vi "GUI_v3.vi"() -> ()   [LabVIEW 2023]
uses:
  Serial - Settings.ctl
  <vilib>/Utility/miscctls.llb/LVRGBAColorTypeDef.ctl
  <vilib>/Utility/miscctls.llb/LV3DPointTypeDef.ctl
  e2109eba-4716-5941-afb7-b0faa504542a.vi
  327bca25-9371-1e41-8126-f95c64e27f6d.vi
  abf5b892-6ba6-6f43-be19-45be42e399fc.vi
  44eb8c8b-3870-a84c-bb75-4112acaa9c04.vi
  f7abd40d-e190-3443-8a30-185c2517432b.vi
  <vilib>/Array/Sort 2D Array - Pop Stack.vi
  <vilib>/Array/Sort 2D Array - Push Stack.vi
  327bca25-9371-1e41-8126-f95c64e27f6d.vi/269d4b3b-47f5-49e3-8884-44851e4dd9d5.vi
  327bca25-9371-1e41-8126-f95c64e27f6d.vi/6d99389c-673d-4efb-bf33-19b32bcf4cf8.vi
  abf5b892-6ba6-6f43-be19-45be42e399fc.vi/269d4b3b-47f5-49e3-8884-44851e4dd9d5.vi
  abf5b892-6ba6-6f43-be19-45be42e399fc.vi/6d99389c-673d-4efb-bf33-19b32bcf4cf8.vi
  44eb8c8b-3870-a84c-bb75-4112acaa9c04.vi/269d4b3b-47f5-49e3-8884-44851e4dd9d5.vi
  44eb8c8b-3870-a84c-bb75-4112acaa9c04.vi/6d99389c-673d-4efb-bf33-19b32bcf4cf8.vi
  f7abd40d-e190-3443-8a30-185c2517432b.vi/269d4b3b-47f5-49e3-8884-44851e4dd9d5.vi
  f7abd40d-e190-3443-8a30-185c2517432b.vi/6d99389c-673d-4efb-bf33-19b32bcf4cf8.vi
  <vilib>/Instr/_visa.llb/VISA Configure Serial Port (Instr).vi
  <vilib>/picture/3D Picture Control/Object/Create Object (drawable).vi
  <vilib>/picture/3D Picture Control/Object/Add Object (no reference).vi
  <vilib>/picture/3D Picture Control/NI_3D Picture Control.lvlib
panel:
  out "read buffer":string
  out "output string":string
  in  "X":bool
  in  "Y":bool
  in  "Z":bool
  in  "[ESC]":bool
  out "Buffer length":i32
  in  "Serial Settings":T1={"baud rate"=115200, "data bits"=8, "parity"=enum."None", "stop bits"=10, "flow control"=0} {"flow control" items=["None"=0, "XON/XOFF"=1, "RTS/CTS"=2, "DTR/DSR"=4]; "stop bits" items=["1.0"=10, "1.5"=15, "2.0"=20]; "data bits" min=5 max=8 step=1; "baud rate" items=["75"=75, "110"=110, "134"=134, "150"=150, "300"=300, "600"=600, "1200"=1200, "1800"=1800, "2400"=2400, "4800"=4800, "7200"=7200, "9600"=9600, "14400"=14400, "19200"=19200, "28800"=28800, "38400"=38400, "56000"=56000, "57600"=57600, "115200"=115200, "128000"=128000, "230400"=230400]}
  out "Input length":i32
  in  "Draw Mode":T2(ring)
  in  "Front":bool
  out "3D Picture":refnum<vi>(3d-picture)
  out "Number of Points":i32
  in  "Clear":bool
  in  "From File?":bool
  in  "File path":path
  in  "VISA resource name":refnum<visa-resource-name>
  in  "Back":bool
  in  "Up":bool
  in  "Down":bool
  in  "Right":bool
  in  "Left":bool
  # "3D LED HOLOGRAM\n1. Enter VISA resource name\n2. Import a file\n3. Run the program"
  # "FIVE GUYS"
  # "Import File"
  # "TRANSLATION"
  # "X"
  # "Y"
  # "Z"
  # "ROTATION"
  # "X"
  # "Y"
  # "Z"
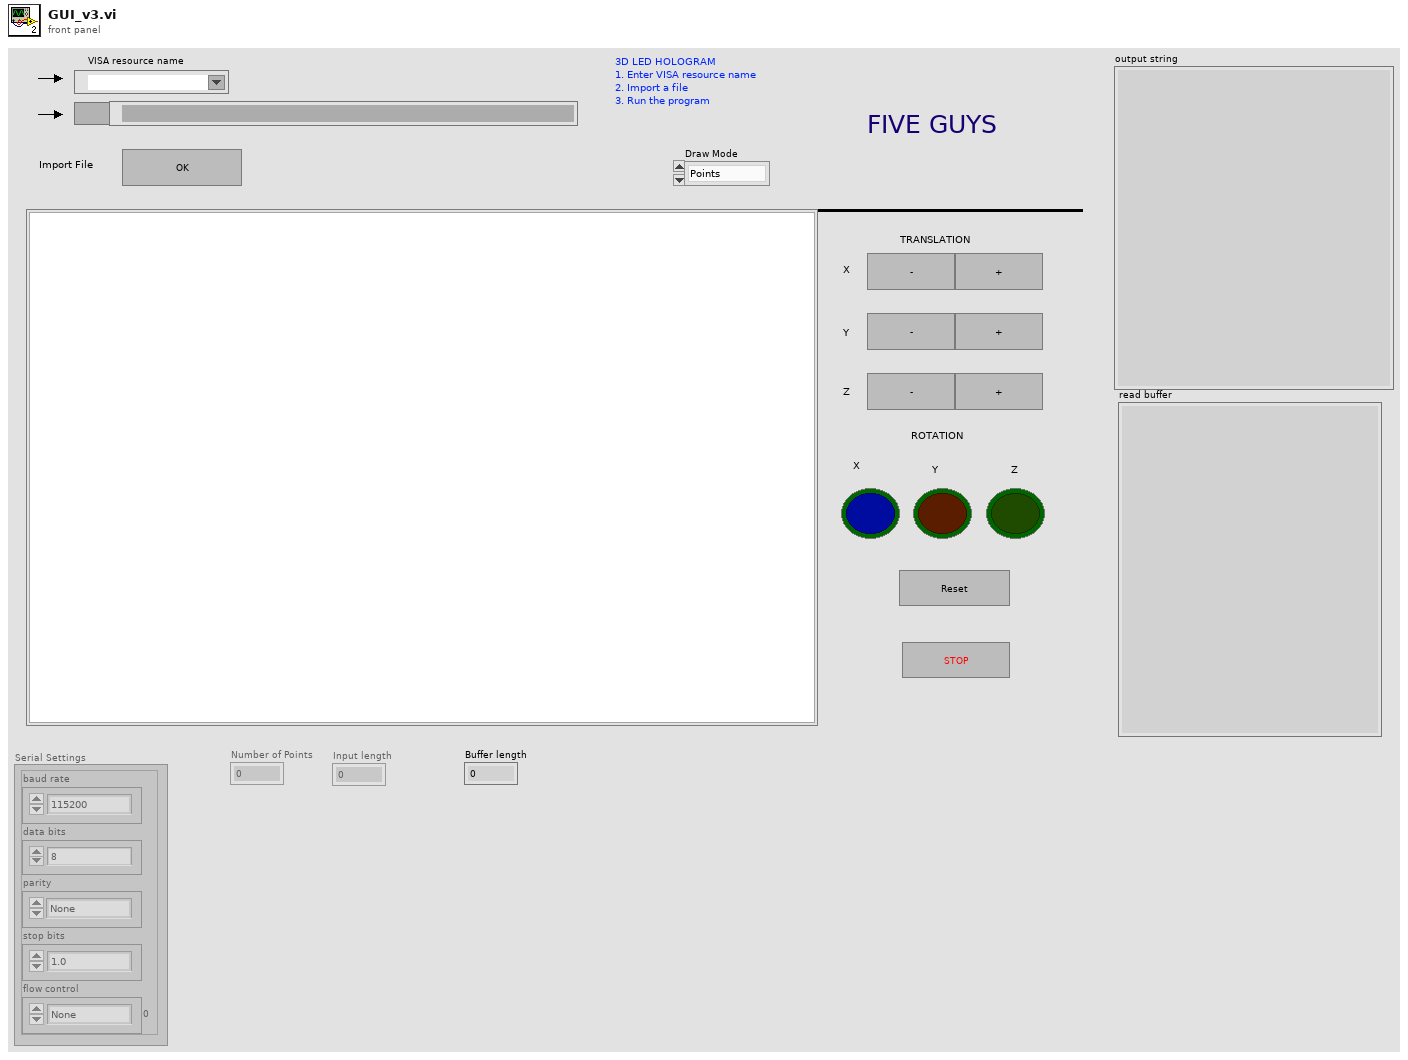
[diagram p1: front panel]
types:
  T1 = typedef "Serial - Settings.ctl" = cluster{"baud rate":u32, "data bits":u16, "parity":enum16{"None", "Odd", "Even", "Mark", "Space"}, "stop bits":u16, "flow control":u16}
  T2 = enum16{"Points", "Lines", "Line Strip", "Line Loop", "Triangles", "Triangle Strip", "Triangle Fan", "Quads", "Quad Strip", "Polygon"}
  T3 = typedef "LVRGBAColorTypeDef.ctl" = cluster{"Red":sgl, "Green":sgl, "Blue":sgl, "Alpha":sgl}
  T4 = enum16{"Overall", "Per Primitive", "Per Vertex", "Binding Off"}
  T5 = cluster{"Red":sgl, "Green":sgl, "Blue":sgl, "Alpha":sgl}
  T6 = typedef "LV3DPointTypeDef.ctl" = cluster{"X":sgl, "Y":sgl, "Z":sgl}
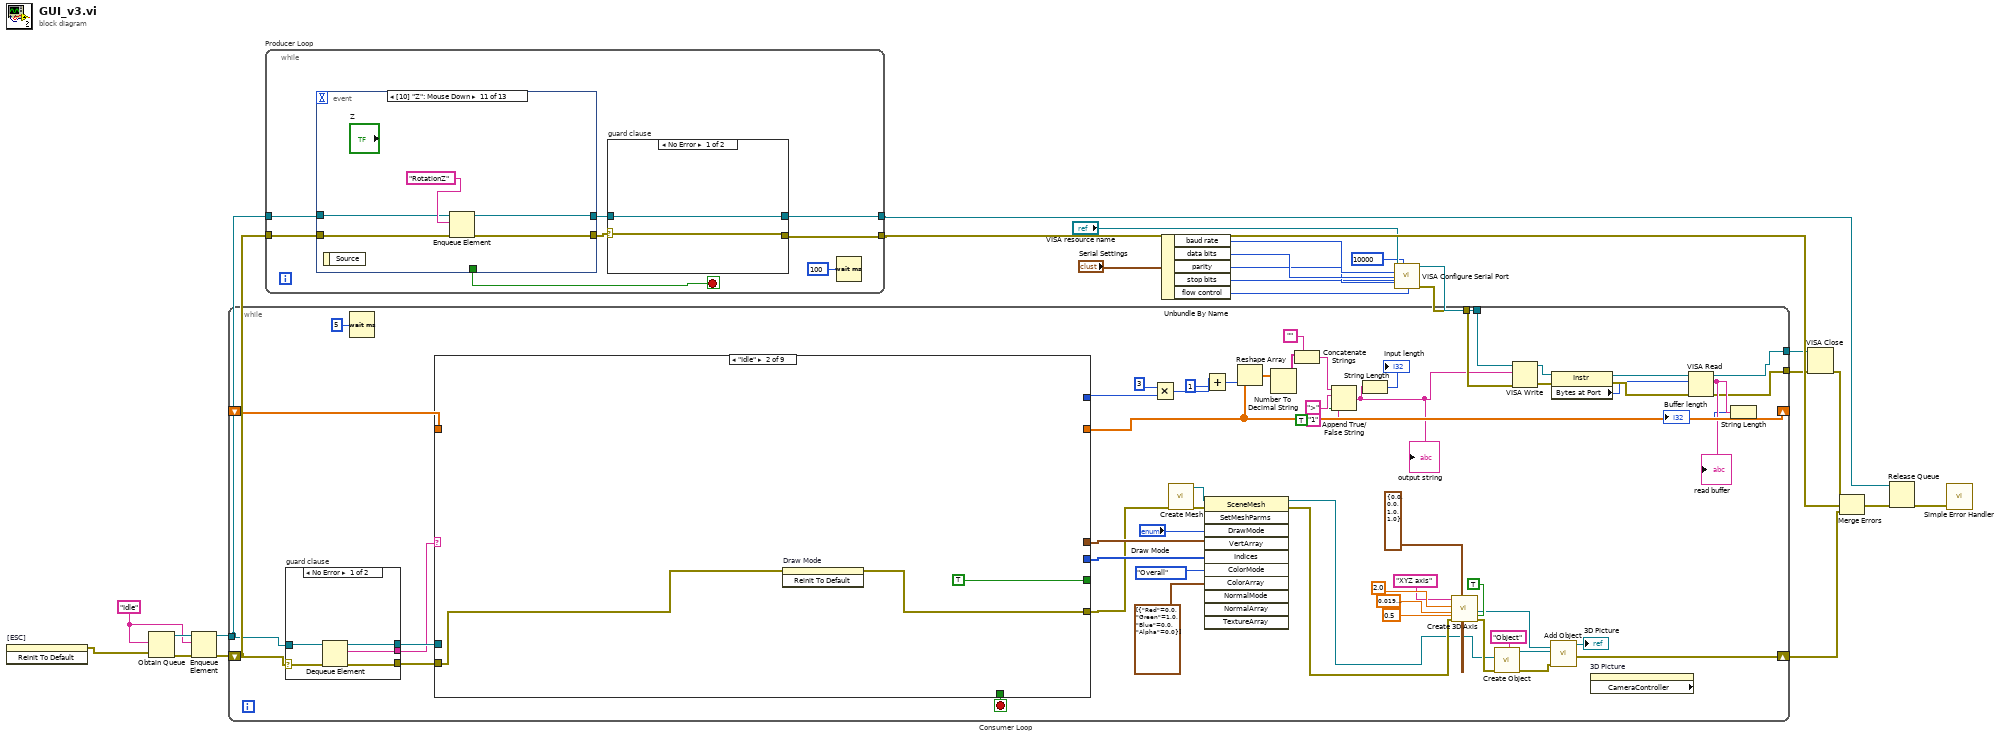
[diagram p0: block diagram]
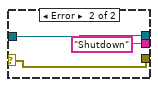
[diagram p2: hidden frame]
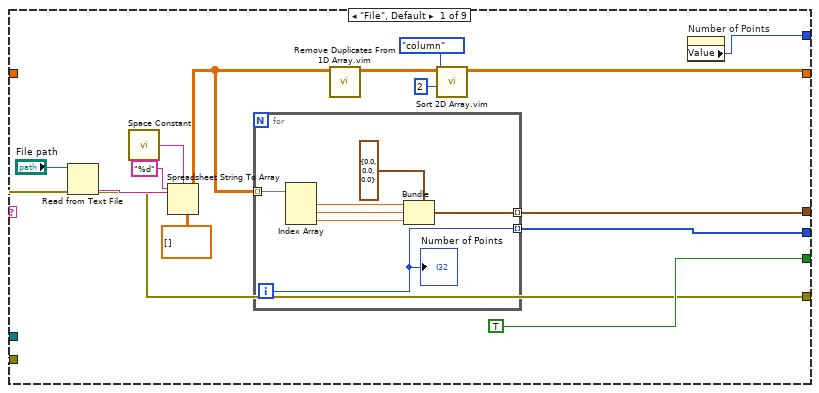
[diagram p3: hidden frame]
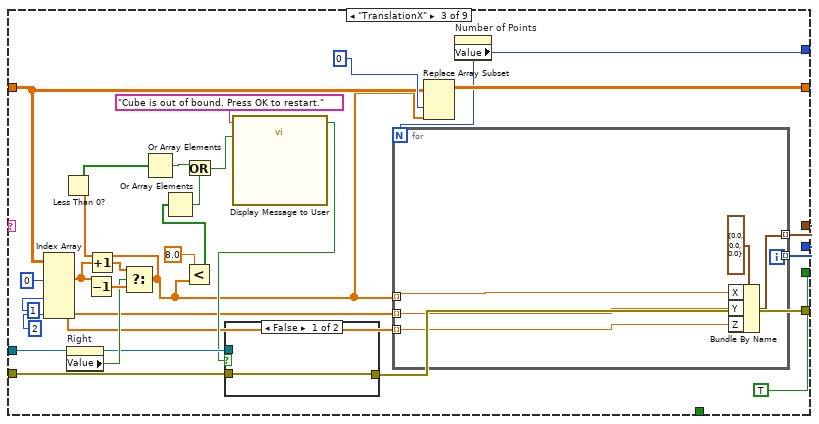
[diagram p4: hidden frame]
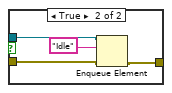
[diagram p5: hidden frame]
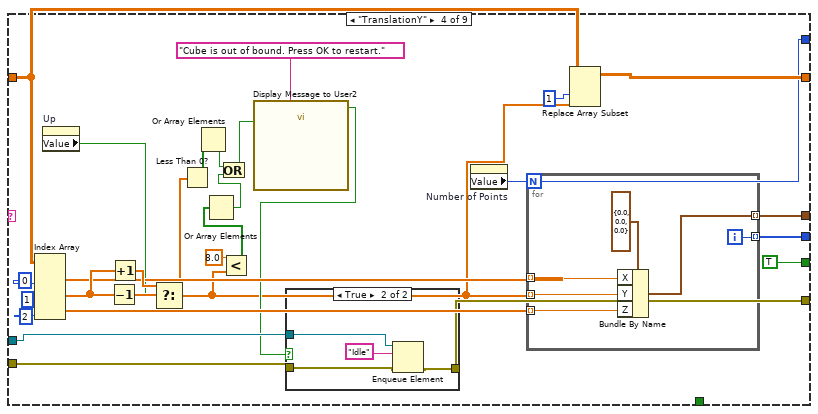
[diagram p6: hidden frame]
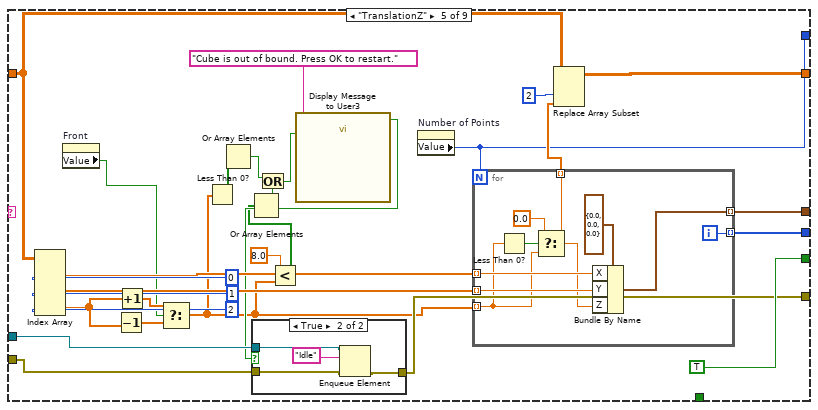
[diagram p8: hidden frame]
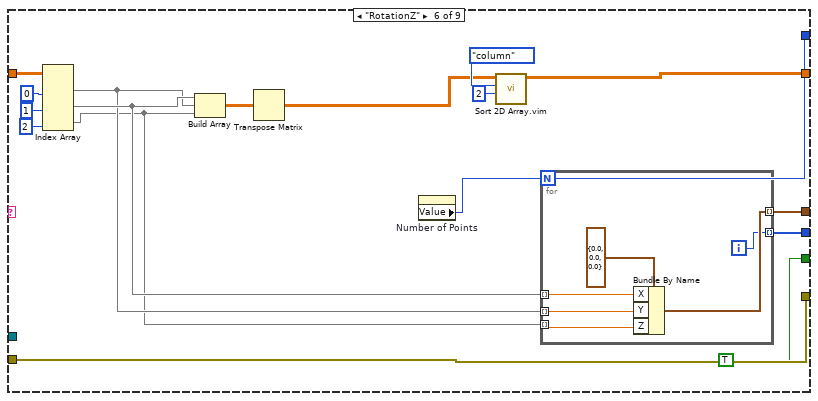
[diagram p10: hidden frame]
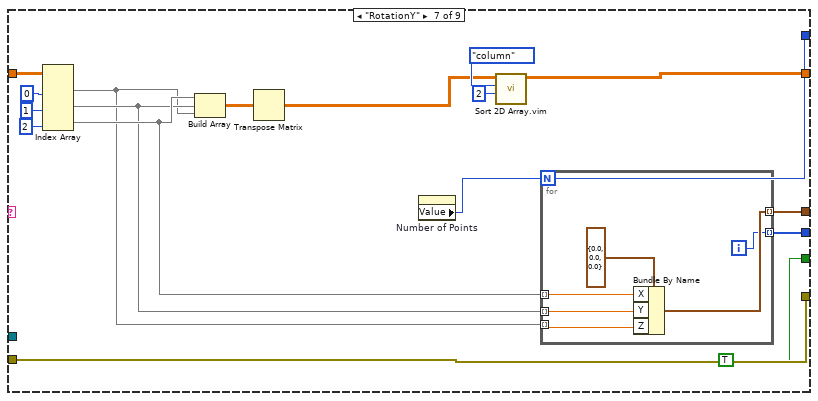
[diagram p11: hidden frame]
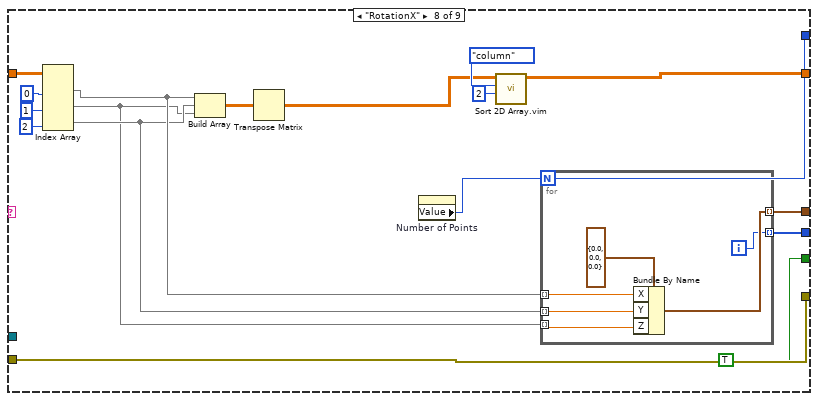
[diagram p12: hidden frame]
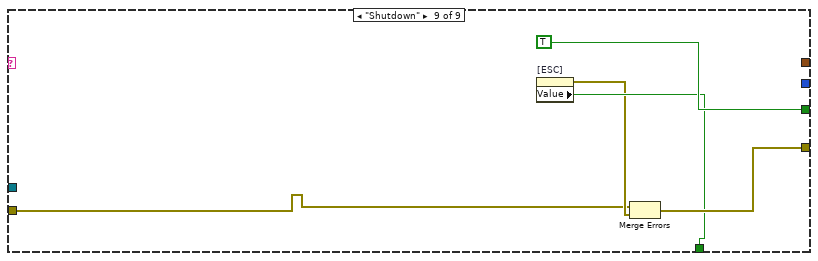
[diagram p13: hidden frame]
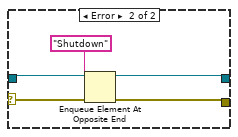
[diagram p14: hidden frame]
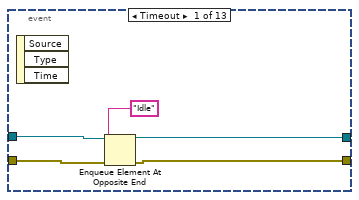
[diagram p15: hidden frame]
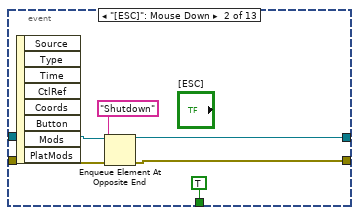
[diagram p16: hidden frame]
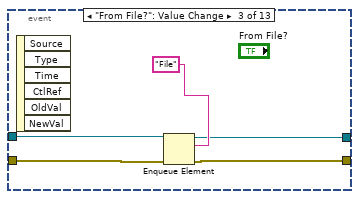
[diagram p17: hidden frame]
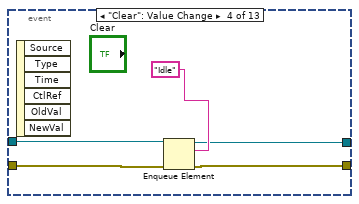
[diagram p18: hidden frame]
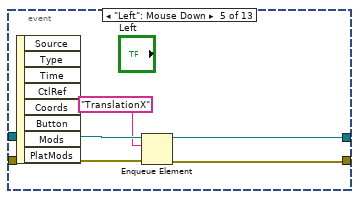
[diagram p19: hidden frame]
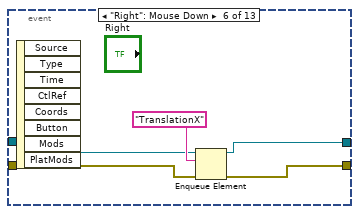
[diagram p20: hidden frame]
diagram:
  w22 = "Idle"
  n1 = invoke on="[ESC]" class="Bool (strict)" method="Reinit To Default"() -> (error out=w1:errorcluster)  [unwired: 3 in, 2 out]
  n2 = Obtain Queue(element data type=w22, error in (no error)=w1) -> (queue out=w23:refnum<queue>, error out=w24:errorcluster)  [unwired: 3 in, 1 out]
  n3 = Enqueue Element(queue=w23, element=w22, error in (no error)=w24) -> (queue out=w21:refnum<queue>, error out=w20:errorcluster)  [unwired: 1 in, 1 out]
  n4 = while "Producer Loop" {
    tunnel: [w28] -> w17
    tunnel: [w27] -> w19
    tunnel: w21 -> [w32]
    tunnel: w20 -> [w31]
    stop <- w26 stop-if-true
    n5 = event shown="[10] \"Z\": Mouse Down" {
      selector: _ -> [_ _ _ _ _ _ _ _ _ _ _ _ _]
      dyn-events: _ -> [_ _ _ _ _ _ _ _ _ _ _ _ _]
      timeout: _ -> [_ _ _ _ _ _ _ _ _ _ _ _ _]
      tunnel: [_ TRUE ("[ESC]") _ _ _ _ _ _ _ _ _ _ _] -> w26
      tunnel: [w43 w49 w51 w56 w61 w66 w71 w76 w81 w86 w94 w99 w104] -> w29
      tunnel: [w42 w48 w52 w57 w64 w67 w72 w77 w82 w87 w93 w98 w103] -> w30
      tunnel: w32 -> [w41 w47 w53 w58 w65 w69 w74 w79 w84 w89 w92 w97 w102]
      tunnel: w31 -> [w40 w46 w54 w59 w63 w68 w73 w78 w83 w88 w91 w96 w101]
      event Timeout {
        n6 = event-data() -> ()  [unwired: 1 in, 3 out]
        n7 = Enqueue Element At Opposite End(queue=w41, element="Idle", error in (no error)=w40) -> (queue out=w42:refnum<queue>, error out=w43:errorcluster)  [unwired: 1 in, 1 out]
      }
      event "[ESC]": Mouse Down {
        n8 = event-data() -> ()  [unwired: 1 in, 8 out]
        n9 = Enqueue Element At Opposite End(queue=w47, element="Shutdown", error in (no error)=w46) -> (queue out=w48:refnum<queue>, error out=w49:errorcluster)  [unwired: 1 in, 1 out]
      }
      event "From File?": Value Change {
        n10 = event-data() -> ()  [unwired: 1 in, 6 out]
        n11 = Enqueue Element(queue=w53, element="File", error in (no error)=w54) -> (queue out=w52:refnum<queue>, error out=w51:errorcluster)  [unwired: 1 in, 1 out]
      }
      event "Clear": Value Change {
        n12 = event-data() -> ()  [unwired: 1 in, 6 out]
        n13 = Enqueue Element(queue=w58, element="Idle", error in (no error)=w59) -> (queue out=w57:refnum<queue>, error out=w56:errorcluster)  [unwired: 1 in, 1 out]
      }
      event "Left": Mouse Down {
        n14 = event-data() -> ()  [unwired: 1 in, 8 out]
        n15 = Enqueue Element(queue=w65, element="TranslationX", error in (no error)=w63) -> (queue out=w64:refnum<queue>, error out=w61:errorcluster)  [unwired: 1 in, 1 out]
      }
      event "Right": Mouse Down {
        n16 = event-data() -> ()  [unwired: 1 in, 8 out]
        n17 = Enqueue Element(queue=w69, element="TranslationX", error in (no error)=w68) -> (queue out=w67:refnum<queue>, error out=w66:errorcluster)  [unwired: 1 in, 1 out]
      }
      event "Back": Mouse Down {
        n18 = event-data() -> ()  [unwired: 1 in, 8 out]
        n19 = Enqueue Element(queue=w74, element="TranslationZ", error in (no error)=w73) -> (queue out=w72:refnum<queue>, error out=w71:errorcluster)  [unwired: 1 in, 1 out]
      }
      event "Front": Mouse Down {
        n20 = event-data() -> ()  [unwired: 1 in, 8 out]
        n21 = Enqueue Element(queue=w79, element="TranslationZ", error in (no error)=w78) -> (queue out=w77:refnum<queue>, error out=w76:errorcluster)  [unwired: 1 in, 1 out]
      }
      event "Down": Mouse Down {
        n22 = event-data() -> ()  [unwired: 1 in, 8 out]
        n23 = Enqueue Element(queue=w84, element="TranslationY", error in (no error)=w83) -> (queue out=w82:refnum<queue>, error out=w81:errorcluster)  [unwired: 1 in, 1 out]
      }
      event "Up": Mouse Down {
        n24 = event-data() -> ()  [unwired: 1 in, 8 out]
        n25 = Enqueue Element(queue=w89, element="TranslationY", error in (no error)=w88) -> (queue out=w87:refnum<queue>, error out=w86:errorcluster)  [unwired: 1 in, 1 out]
      }
      event "Z": Mouse Down {
        n26 = event-data() -> ()  [unwired: 1 in, 1 out]
        n27 = Enqueue Element(queue=w92, element="RotationZ", error in (no error)=w91) -> (queue out=w93:refnum<queue>, error out=w94:errorcluster)  [unwired: 1 in, 1 out]
      }
      event "Y": Mouse Down {
        n28 = event-data() -> ()  [unwired: 1 in, 1 out]
        n29 = Enqueue Element(queue=w97, element="RotationY", error in (no error)=w96) -> (queue out=w98:refnum<queue>, error out=w99:errorcluster)  [unwired: 1 in, 1 out]
      }
      event "X": Mouse Down {
        n30 = event-data() -> ()  [unwired: 1 in, 1 out]
        n31 = Enqueue Element(queue=w102, element="RotationX", error in (no error)=w101) -> (queue out=w103:refnum<queue>, error out=w104:errorcluster)  [unwired: 1 in, 1 out]
      }
    }
    n32 = case "guard clause" shown="No Error" w29 {
      selector: w29 -> [w33 w38]
      tunnel: w30 -> [w34 w39]
      tunnel: [w34 w36] -> w28
      tunnel: [w33 w37] -> w27
      frame No Error {
      }
      frame Error {
        n33 = Enqueue Element At Opposite End(queue=w39, element="Shutdown", error in (no error)=w38) -> (queue out=w36:refnum<queue>, error out=w37:errorcluster)  [unwired: 1 in, 1 out]
      }
    }
    n34 = Wait (ms)(milliseconds to wait=u32 100) -> ()  [unwired: 1 out]
  }
  n35 = Unbundle By Name("Serial Settings") -> ("baud rate"=w10:u32, "data bits"=w9:u16, "parity"=w8:enum16{"None", "Odd", "Even", "Mark", "Space"}, "stop bits"=w7:u16, "flow control"=w6:u16)
  n36 = call-poly "VISA Configure Serial Port"("VISA resource name"="VISA resource name", "timeout (10sec)"=u32 10000, "baud rate (9600)"=w10, "data bits (8)"=w9, "parity (0:none)"=w8, "stop bits (10: 1 bit)"=w7, "flow control (0:none)"=w6) -> ("VISA resource name out"=w5:refnum<visa-resource-name>, "error out"=w4:errorcluster)  [unwired: 7 in]
  n37 = while "Consumer Loop" {
    tunnel: w21 -> [w162]
    shift-right: [w135] -> w16
    shift-left: w20 -> [w159]
    shift-right: [w134] -> _
    shift-left: _ -> [w156]
    tunnel: w5 -> [w144]
    tunnel: w4 -> [w143]
    tunnel: [w106] -> w15
    tunnel: [w107] -> w14
    stop <- w160 stop-if-true
    n38 = case "guard clause" shown="No Error" w159 {
      selector: w159 -> [w166 w169]
      tunnel: w162 -> [w167 w170]
      tunnel: [w165 w169] -> w161
      tunnel: [w164 "Shutdown"] -> w117
      tunnel: [w163 w170] -> w142
      frame No Error {
        n39 = Dequeue Element(queue=w167, error in (no error)=w166) -> (queue out=w163:refnum<queue>, element=w164:string, error out=w165:errorcluster)  [unwired: 1 in, 1 out]
      }
      frame Error {
      }
    }
    n40 = Wait (ms)(milliseconds to wait=u32 5) -> ()  [unwired: 1 out]
    n41 = case shown="\"Idle\"" w117 {
      tunnel: w161 -> [w178 w195 w209 w245 w287 w334 w357 w380 w387]
      tunnel: w142 -> [_ _ w210 w246 w288 _ _ _ _]
      tunnel: [_ _ _ _ _ _ _ _ w389] -> w160
      tunnel: [w177 w194 w208 w244 w286 w334 w357 w380 w391] -> w155
      tunnel: [w185 _ w219 w256 w296 w325 w348 w371 _] -> w158
      tunnel: [w184 _ w218 w255 w295 w324 w347 w370 _] -> w157
      tunnel: [TRUE TRUE TRUE TRUE TRUE TRUE TRUE TRUE TRUE] -> _
      tunnel: [w174 _ w214 w262 w302 w323 w346 w369 _] -> w134
      tunnel: w156 -> [_ _ w223 w261 w301 w330 w353 w376 _]
      tunnel: [w171 _ w197 w236 w275 w318 w341 w364 _] -> w113
      frame "File", Default {
        n42 = Read from Text File(file (use dialog)="File path", error in=w178) -> (text=w182:string, error out=w177:errorcluster)  [unwired: 2 in, 2 out]
        n43 = call <vilib>:"Space Constant.vi"() -> ("String"=w181:string)
        n44 = Spreadsheet String To Array(delimiter (Tab)=w181, format string="%d", spreadsheet string=w182, array type (2D Dbl)=sgl[][] []) -> (array=w176:sgl[][])
        n45 = for {
          tunnel: w176 -> [w187] mode=indexing
          tunnel: [w189] -> w185 mode=indexing
          tunnel: [w188] -> w184 mode=indexing
          i -> [w188]
          n46 = Index Array(array=w187) -> (element #1=w192:sgl, element #2=w191:sgl, element #3=w190:sgl)  [unwired: 3 in]
          n47 = Bundle(cluster=T6 {"X"=0.0, "Y"=0.0, "Z"=0.0} ("3D Point"), "X"=w192, "Y"=w191, "Z"=w190) -> (w189:T6)
          "Number of Points" <- w188
        }
        n48 = call "Remove Duplicates From 1D Array.vim"("array"=w176) -> ("array with duplicates removed"=w175:sgl[][])  [unwired: 10 in]
        n49 = call "Sort 2D Array.vim"("index"=2, "dimension to index (column)"=enum16{"column", "row"}."column", "2D array"=w175) -> ("sorted 2D array"=w174:sgl[][])  [unwired: 7 in, 1 out]
        n50 = property on="Number of Points" class="DigNum (strict)"() -> ("Value"=w171:i32)  [unwired: 2 in, 2 out]
      }
      frame "Idle" {
        n51 = invoke on="Draw Mode" class="Enum (strict)" method="Reinit To Default"(error in=w195) -> (error out=w194:errorcluster)  [unwired: 2 in, 2 out]
      }
      frame "TranslationX" {
        n52 = Index Array(array=w223, index (col) #1=0 ("disabled index (col)"), index (col) #2=1 ("index (col)"), index (col) #3=2 ("index (col)")) -> (element #1=w200:dbl[], element #2=w199:dbl[], element #3=w198:dbl[])  [unwired: 3 in]
        n53 = property on="Right" class="Bool (strict)"() -> ("Value"=w215:bool)  [unwired: 2 in, 2 out]
        n54 = Decrement(x=w200) -> (x-1=w217:dbl[])
        n55 = Increment(x=w200) -> (x+1=w216:dbl[])
        n56 = Select(t=w216, s=w215, f=w217) -> (s? t:f=w201:dbl[])
        n57 = Less Than 0?(x=w201) -> (x < 0?=w212:bool[])
        n58 = Or Array Elements(Boolean array=w212) -> (logical OR=w205:bool)
        n59 = Less?(x=8.0, y=w201) -> (x < y?=w202:bool[])
        n60 = Or Array Elements(Boolean array=w202) -> (logical OR=w206:bool)
        n61 = Or(x=w205, y=w206) -> (x .or. y?=w204:bool)
        n62 = call "Display Message to User"("Enable"=w204, "Message"="Cube is out of bound. Press OK to restart.") -> ("OK"=w207:bool)  [unwired: 8 in, 1 out]
        n63 = case shown="False" w207 {
          tunnel: w210 -> [_ w227]
          tunnel: w209 -> [w225 w229]
          tunnel: [w225 w228] -> w208
          frame False {
          }
          frame True {
            n64 = Enqueue Element(queue=w227, element="Idle", error in (no error)=w229) -> (error out=w228:errorcluster)  [unwired: 1 in, 2 out]
          }
        }
        n65 = Replace Array Subset(array=w223, new element=w201, index (col)=0 ("disabled index (col)")) -> (w214:dbl[][])  [unwired: 1 in]
        n66 = property on="Number of Points" class="DigNum (strict)"() -> ("Value"=w197:i32)  [unwired: 2 in, 2 out]
        n67 = for {
          N: w197 -> [_]
          tunnel: w201 -> [w230] mode=indexing
          tunnel: w199 -> [w235] mode=indexing
          tunnel: w198 -> [w234] mode=indexing
          tunnel: [w233] -> w219 mode=indexing
          tunnel: [w231] -> w218 mode=indexing
          i -> [w231]
          n68 = Bundle By Name(cluster=T6 {"X"=0.0, "Y"=0.0, "Z"=0.0} ("3D Point"), "X"=w230, "Y"=w235, "Z"=w234) -> (w233:T6)
        }
      }
      frame "TranslationY" {
        n69 = Index Array "Index Array"(array=w261, index (col) #1=0 ("disabled index (col)"), index (col) #2=1 ("index (col)"), index (col) #3=2 ("index (col)")) -> (element #1=w251:dbl[], element #2=w252:dbl[], element #3=w257:dbl[])  [unwired: 3 in]
        n70 = property on="Up" class="Bool (strict)"() -> ("Value"=w250:bool)  [unwired: 2 in, 2 out]
        n71 = Decrement(x=w252) -> (x-1=w254:dbl[])
        n72 = Increment(x=w252) -> (x+1=w253:dbl[])
        n73 = Select(t=w253, s=w250, f=w254) -> (s? t:f=w237:dbl[])
        n74 = Less Than 0?(x=w237) -> (x < 0?=w248:bool[])
        n75 = Or Array Elements(Boolean array=w248) -> (logical OR=w240:bool)
        n76 = Less?(x=8.0, y=w237) -> (x < y?=w241:bool[])
        n77 = Or Array Elements(Boolean array=w241) -> (logical OR=w239:bool)
        n78 = Or(x=w240, y=w239) -> (x .or. y?=w238:bool)
        n79 = call "Display Message to User2"("Enable"=w238, "Message"="Cube is out of bound. Press OK to restart.") -> ("OK"=w243:bool)  [unwired: 8 in, 1 out]
        n80 = case shown="True" w243 {
          tunnel: w245 -> [w264 w268]
          tunnel: [w264 w267] -> w244
          tunnel: w246 -> [_ w265]
          frame False {
          }
          frame True {
            n81 = Enqueue Element(queue=w265, element="Idle", error in (no error)=w268) -> (error out=w267:errorcluster)  [unwired: 1 in, 2 out]
          }
        }
        n82 = property on="Number of Points" class="DigNum (strict)"() -> ("Value"=w236:i32)  [unwired: 2 in, 2 out]
        n83 = for {
          N: w236 -> [_]
          tunnel: w251 -> [w274] mode=indexing
          tunnel: w237 -> [w269] mode=indexing
          tunnel: w257 -> [w273] mode=indexing
          tunnel: [w272] -> w256 mode=indexing
          tunnel: [w270] -> w255 mode=indexing
          i -> [w270]
          n84 = Bundle By Name(cluster=T6 {"X"=0.0, "Y"=0.0, "Z"=0.0} ("3D Point"), "X"=w274, "Y"=w269, "Z"=w273) -> (w272:T6)
        }
        n85 = Replace Array Subset(array=w261, new element=w237, index (col)=1 ("disabled index (col)")) -> (w262:dbl[][])  [unwired: 1 in]
      }
      frame "TranslationZ" {
        n86 = Index Array "Index Array"(array=w301, index (col) #1=0 ("disabled index (col)"), index (col) #2=1 ("index (col)"), index (col) #3=2 ("index (col)")) -> (element #1=w291:dbl[], element #2=w297:dbl[], element #3=w292:dbl[])  [unwired: 3 in]
        n87 = property on="Front" class="Bool (strict)"() -> ("Value"=w283:bool)  [unwired: 2 in, 2 out]
        n88 = Decrement(x=w292) -> (x-1=w294:dbl[])
        n89 = Increment(x=w292) -> (x+1=w293:dbl[])
        n90 = Select(t=w293, s=w283, f=w294) -> (s? t:f=w279:dbl[])
        n91 = Less Than 0?(x=w279) -> (x < 0?=w285:bool[])
        n92 = Or Array Elements(Boolean array=w285) -> (logical OR=w277:bool)
        n93 = Less?(x=8.0, y=w279) -> (x < y?=w280:bool[])
        n94 = Or Array Elements(Boolean array=w280) -> (logical OR=w278:bool)
        n95 = Or(x=w277, y=w278) -> (x .or. y?=w276:bool)
        n96 = call "Display Message to User3"("Enable"=w276, "Message"="Cube is out of bound. Press OK to restart.") -> ("OK"=w282:bool)  [unwired: 8 in, 1 out]
        n97 = case shown="True" w282 {
          tunnel: w288 -> [_ w306]
          tunnel: w287 -> [w304 w308]
          tunnel: [w304 w307] -> w286
          frame False {
          }
          frame True {
            n98 = Enqueue Element(queue=w306, element="Idle", error in (no error)=w308) -> (error out=w307:errorcluster)  [unwired: 1 in, 2 out]
          }
        }
        n99 = property on="Number of Points" class="DigNum (strict)"() -> ("Value"=w275:i32)  [unwired: 2 in, 2 out]
        n100 = for {
          N: w275 -> [_]
          tunnel: w291 -> [w317] mode=indexing
          tunnel: w297 -> [w316] mode=indexing
          tunnel: w279 -> [w309] mode=indexing
          tunnel: [w315] -> w296 mode=indexing
          tunnel: [w313] -> w295 mode=indexing
          tunnel: [w310] -> w289 mode=indexing
          i -> [w313]
          n101 = Less Than 0?(x=w309) -> (x < 0?=w312:bool)
          n102 = Select(t=0.0, s=w312, f=w309) -> (s? t:f=w310:dbl)
          n103 = Bundle By Name(cluster=T6 {"X"=0.0, "Y"=0.0, "Z"=0.0} ("3D Point"), "X"=w317, "Y"=w316, "Z"=w310) -> (w315:T6)
        }
        n104 = Replace Array Subset(array=w301, new element=w289, index (col)=2 ("disabled index (col)")) -> (w302:dbl[][])  [unwired: 1 in]
      }
      frame "RotationZ" {
        n105 = Index Array "Index Array"(array=w330, index (col) #1=0 ("disabled index (col)"), index (col) #2=1 ("index (col)"), index (col) #3=2 ("index (col)")) -> (element #1=w320:dbl[], element #2=w321:dbl[], element #3=w319:dbl[])  [unwired: 3 in]
        n106 = Build Array(w321, w320, w319) -> (w329:dbl[][])
        n107 = Transpose Matrix(1:w329) -> (0:w322:dbl[][])
        n108 = property on="Number of Points" class="DigNum (strict)"() -> ("Value"=w318:i32)  [unwired: 2 in, 2 out]
        n109 = call "Sort 2D Array.vim"("index"=2, "dimension to index (column)"=enum16{"column", "row"}."column", "2D array"=w322) -> ("sorted 2D array"=w323:dbl[][])  [unwired: 7 in, 1 out]
        n110 = for {
          N: w318 -> [_]
          tunnel: w321 -> [w339] mode=indexing
          tunnel: w320 -> [w338] mode=indexing
          tunnel: w319 -> [w337] mode=indexing
          tunnel: [w336] -> w325 mode=indexing
          tunnel: [w335] -> w324 mode=indexing
          i -> [w335]
          n111 = Bundle By Name(cluster=T6 {"X"=0.0, "Y"=0.0, "Z"=0.0} ("3D Point"), "X"=w339, "Y"=w338, "Z"=w337) -> (w336:T6)
        }
      }
      frame "RotationY" {
        n112 = Index Array "Index Array"(array=w353, index (col) #1=0 ("disabled index (col)"), index (col) #2=1 ("index (col)"), index (col) #3=2 ("index (col)")) -> (element #1=w342:dbl[], element #2=w343:dbl[], element #3=w344:dbl[])  [unwired: 3 in]
        n113 = Build Array(w344, w343, w342) -> (w352:dbl[][])
        n114 = Transpose Matrix(1:w352) -> (0:w345:dbl[][])
        n115 = property on="Number of Points" class="DigNum (strict)"() -> ("Value"=w341:i32)  [unwired: 2 in, 2 out]
        n116 = call "Sort 2D Array.vim"("index"=2, "dimension to index (column)"=enum16{"column", "row"}."column", "2D array"=w345) -> ("sorted 2D array"=w346:dbl[][])  [unwired: 7 in, 1 out]
        n117 = for {
          N: w341 -> [_]
          tunnel: w344 -> [w362] mode=indexing
          tunnel: w343 -> [w361] mode=indexing
          tunnel: w342 -> [w360] mode=indexing
          tunnel: [w359] -> w348 mode=indexing
          tunnel: [w358] -> w347 mode=indexing
          i -> [w358]
          n118 = Bundle By Name(cluster=T6 {"X"=0.0, "Y"=0.0, "Z"=0.0} ("3D Point"), "X"=w362, "Y"=w361, "Z"=w360) -> (w359:T6)
        }
      }
      frame "RotationX" {
        n119 = Index Array "Index Array"(array=w376, index (col) #1=0 ("disabled index (col)"), index (col) #2=1 ("index (col)"), index (col) #3=2 ("index (col)")) -> (element #1=w367:dbl[], element #2=w365:dbl[], element #3=w366:dbl[])  [unwired: 3 in]
        n120 = Build Array(w367, w366, w365) -> (w375:dbl[][])
        n121 = Transpose Matrix(1:w375) -> (0:w368:dbl[][])
        n122 = property on="Number of Points" class="DigNum (strict)"() -> ("Value"=w364:i32)  [unwired: 2 in, 2 out]
        n123 = call "Sort 2D Array.vim"("index"=2, "dimension to index (column)"=enum16{"column", "row"}."column", "2D array"=w368) -> ("sorted 2D array"=w369:dbl[][])  [unwired: 7 in, 1 out]
        n124 = for {
          N: w364 -> [_]
          tunnel: w367 -> [w385] mode=indexing
          tunnel: w366 -> [w384] mode=indexing
          tunnel: w365 -> [w383] mode=indexing
          tunnel: [w382] -> w371 mode=indexing
          tunnel: [w381] -> w370 mode=indexing
          i -> [w381]
          n125 = Bundle By Name(cluster=T6 {"X"=0.0, "Y"=0.0, "Z"=0.0} ("3D Point"), "X"=w385, "Y"=w384, "Z"=w383) -> (w382:T6)
        }
      }
      frame "Shutdown" {
        n126 = property on="[ESC]" class="Bool (strict)"() -> (error out=w388:errorcluster, "Value"=w389:bool)  [unwired: 2 in, 1 out]
        n127 = Merge Errors(w387, w388) -> (w391:errorcluster)
      }
    }
    n128 = Multiply(x=3 ("y"), y=w113) -> (x*y=w123:i32)
    n129 = call <vilib>:"Create Mesh.vi"("error in (no error)"=w155) -> ("error out"=w112:errorcluster, "New Mesh Refnum"=w111:refnum<vi>)  [unwired: 9 in]
    n130 = Add(x=w123, y=1) -> (x+y=w124:i32)
    n131 = invoke class="SceneMesh" method="SetMeshParms"(reference=w111, error in=w112, "DrawMode"="Draw Mode", "VertArray"=w158, "Indices"=w157, "ColorMode"=T4."Overall" ("Color Binding Mode"), "ColorArray"=T3[] [{"Red"=0.0, "Green"=1.0, "Blue"=0.0, "Alpha"=0.0}] ("Color Array")) -> (reference out=w137:refnum<vi>, error out=w139:errorcluster)  [unwired: 4 in, 9 out]
    n132 = Reshape Array(w134, w124) -> (w132:dbl[])
    n133 = Number To Decimal String(number=w132) -> (decimal integer string=w118:string[])  [unwired: 1 in]
    n134 = Concatenate Strings(w118, "") -> (w129:string)
    n135 = Append True/False String(1:TRUE ("selector"), 2:"1" ("false string"), 3:">" ("true string"), 4:w129) -> (0:w128:string)
    "output string" <- w128
    n136 = String Length(string=w128) -> (length=→"Input length":i32)
    n137 = call <vilib>:"Create 3D Axis.vi"("Character Size"=sgl 0.5, "Axis label?"=TRUE, "Color"=T5 {"Red"=0.0, "Green"=0.0, "Blue"=1.0, "Alpha"=1.0}, "error in (no error)"=w139, "Radius"=sgl 0.02, "Length"=sgl 2.0, "Name"="XYZ axis") -> ("error out"=w138:errorcluster, "New Object Refnum"=w140:refnum<vi>)  [unwired: 3 in]
    n138 = call-poly <vilib>:"Create Object.vi"("error in (no error)"=w138, "Geometry"=w137, "Name"="Object") -> ("error out"=w136:errorcluster, "Scene:New Object"=w116:refnum<vi>)  [unwired: 7 in]
    n139 = VISA Write(VISA resource name=w144, write buffer=w128, error in (no error)=w143) -> (VISA resource name out=w145:refnum<visa-resource-name>, error out=w147:errorcluster)  [unwired: 1 out]
    n140 = call-poly <vilib>:"Add Object.vi"("error in (no error)"=w136, "New Object In"=w116, "Scene Object In"=w140) -> ("error out"=w135:errorcluster, "Scene Object Out"=→"3D Picture":refnum<vi>)  [unwired: 7 in]
    n141 = property on="Property Node" class="Instr"(reference=w145, error in=w147) -> (reference out=w146:refnum<visa-resource-name>, error out=w148:errorcluster, "Bytes at Port"=w115:u32)
    n142 = property on="3D Picture" class="SceneGraphDisp (strict)" props=["CameraController"]() -> ()  [unwired: 2 in, 3 out]
    n143 = VISA Read(VISA resource name=w146, byte count=w115, error in (no error)=w148) -> (VISA resource name out=w107:refnum<visa-resource-name>, read buffer=w120:string, error out=w106:errorcluster)  [unwired: 1 out]
    "read buffer" <- w120
    n144 = String Length(string=w120) -> (length=→"Buffer length":i32)
  }
  n145 = VISA Close(VISA resource name=w14, error in (no error)=w15) -> (error out=w13:errorcluster)
  n146 = Merge Errors(w13, w19, w16) -> (w18:errorcluster)
  n147 = Release Queue(queue=w17, error in (no error)=w18) -> (error out=w12:errorcluster)  [unwired: 1 in, 2 out]
  n148 = call <vilib>:"Simple Error Handler.vi"("error in (no error)"=w12) -> ()  [unwired: 4 in, 5 out]
